vi "DOportSelector.vi"(8 "I/O element":T1(ring), 11 "value":u8) -> ()   [LabVIEW 2014]
uses:
  <vilib>/rvi/eio/common/nirviEmuTemplateMethod_errors.vi
  <vilib>/eio/EIONode/EIONode.xnode
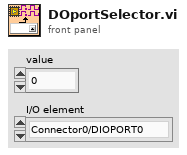
[diagram p1: front panel]
types:
  T1 = enum16{"Connector0/DIOPORT0", "Connector0/DIOPORT1", "Connector1/DIOPORT0", "Connector1/DIOPORT1", "Connector1/DIOPORT2", "Connector1/DIOPORT3", "Connector1/DIOPORT4", "Connector2/DIOPORT0", "Connector2/DIOPORT1", "Connector2/DIOPORT2", "Connector2/DIOPORT3", "Connector2/DIOPORT4"}
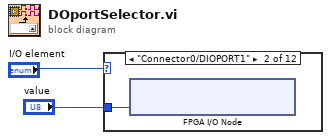
[diagram p0: block diagram]
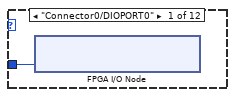
[diagram p2: hidden frame]
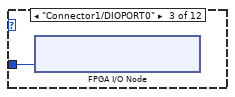
[diagram p3: hidden frame]
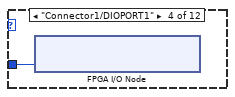
[diagram p4: hidden frame]
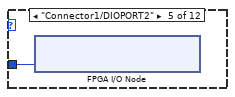
[diagram p5: hidden frame]
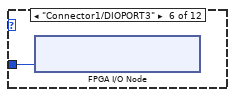
[diagram p6: hidden frame]
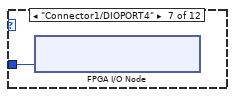
[diagram p7: hidden frame]
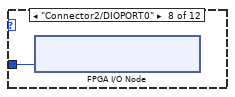
[diagram p8: hidden frame]
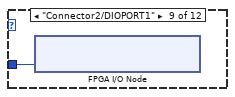
[diagram p9: hidden frame]
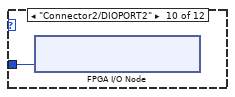
[diagram p10: hidden frame]
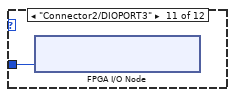
[diagram p11: hidden frame]
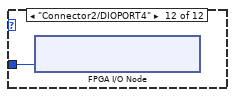
[diagram p12: hidden frame]
diagram:
  n1 = case shown="\"Connector0/DIOPORT1\"" "I/O element" {
    tunnel: "value" -> [w3 w4 w5 w6 w7 w8 w9 w10 w11 w12 w13 w14]
    frame "Connector0/DIOPORT0" {
      n2 = xnode "FPGA I/O Node"("Connector0/DIOPORT0"=w3) -> ()  [unwired: 1 in, 1 out]
    }
    frame "Connector0/DIOPORT1" {
      n3 = xnode "FPGA I/O Node"("Connector0/DIOPORT1"=w4) -> ()  [unwired: 1 in, 1 out]
    }
    frame "Connector1/DIOPORT0" {
      n4 = xnode "FPGA I/O Node"("Connector1/DIOPORT0"=w5) -> ()  [unwired: 1 in, 1 out]
    }
    frame "Connector1/DIOPORT1" {
      n5 = xnode "FPGA I/O Node"("Connector1/DIOPORT1"=w6) -> ()  [unwired: 1 in, 1 out]
    }
    frame "Connector1/DIOPORT2" {
      n6 = xnode "FPGA I/O Node"("Connector1/DIOPORT2"=w7) -> ()  [unwired: 1 in, 1 out]
    }
    frame "Connector1/DIOPORT3" {
      n7 = xnode "FPGA I/O Node"("Connector1/DIOPORT3"=w8) -> ()  [unwired: 1 in, 1 out]
    }
    frame "Connector1/DIOPORT4" {
      n8 = xnode "FPGA I/O Node"("Connector1/DIOPORT4"=w9) -> ()  [unwired: 1 in, 1 out]
    }
    frame "Connector2/DIOPORT0" {
      n9 = xnode "FPGA I/O Node"("Connector2/DIOPORT0"=w10) -> ()  [unwired: 1 in, 1 out]
    }
    frame "Connector2/DIOPORT1" {
      n10 = xnode "FPGA I/O Node"("Connector2/DIOPORT1"=w11) -> ()  [unwired: 1 in, 1 out]
    }
    frame "Connector2/DIOPORT2" {
      n11 = xnode "FPGA I/O Node"("Connector2/DIOPORT2"=w12) -> ()  [unwired: 1 in, 1 out]
    }
    frame "Connector2/DIOPORT3" {
      n12 = xnode "FPGA I/O Node"("Connector2/DIOPORT3"=w13) -> ()  [unwired: 1 in, 1 out]
    }
    frame "Connector2/DIOPORT4" {
      n13 = xnode "FPGA I/O Node"("Connector2/DIOPORT4"=w14) -> ()  [unwired: 1 in, 1 out]
    }
  }
